vi "programa 4 Array.vi"() -> ()   [LabVIEW 2011]
panel:
  out "promedio":dbl
  out "menor":dbl
  out "mayor":dbl
  out "suma":dbl
  out "Array":dbl[](array[numeric])
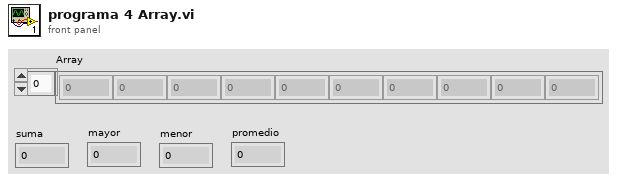
[diagram p1: front panel]
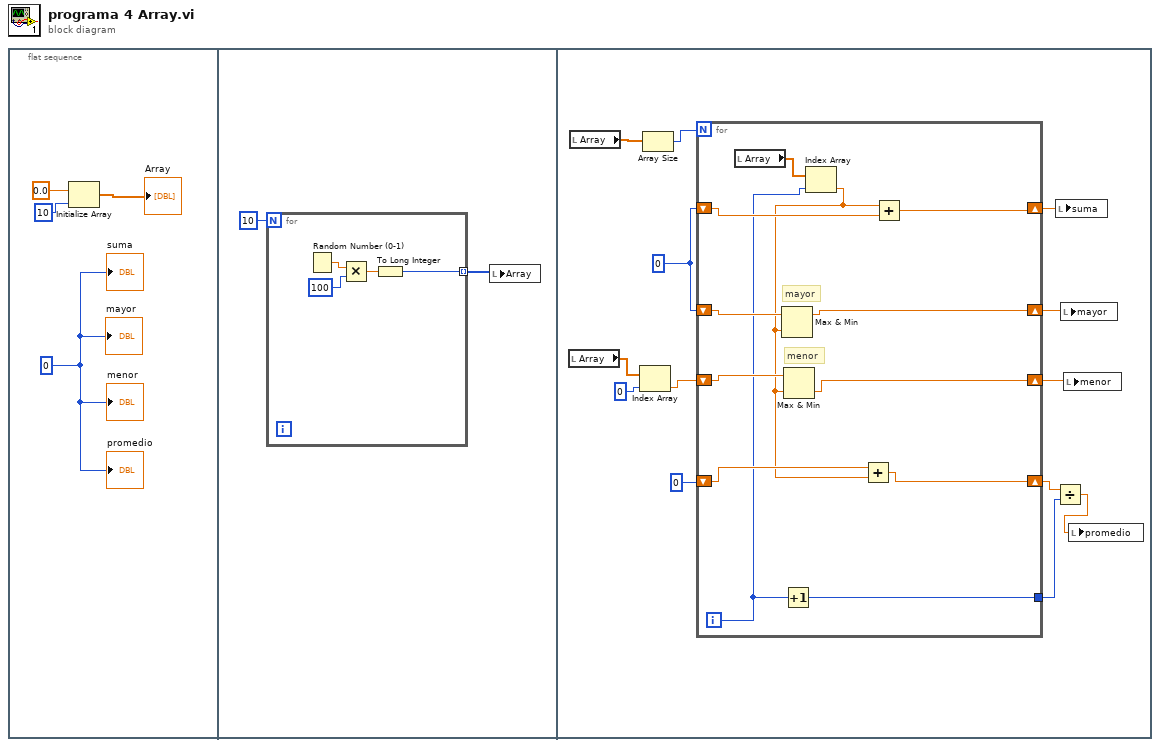
[diagram p0: block diagram]
diagram:
  n1 = flat-sequence {
    frame #0 {
      w1 = 0
      n2 = Initialize Array "Initialize Array"(0.0 ("element"), 10 ("dimension size")) -> (→"Array":dbl[])
      "suma" <- w1
      "mayor" <- w1
      "menor" <- w1
      "promedio" <- w1
    }
    frame #1 {
      n3 = for {
        N: 10 -> [_]
        tunnel: [w7] -> w5 mode=indexing
        n4 = Random Number (0-1)() -> (number: 0 to 1=w10:dbl)
        n5 = Multiply(x=w10, y=100) -> (x*y=w8:dbl)
        n6 = To Long Integer(number=w8) -> (32bit integer=w7:i32)
      }
      n7 = local write "Array"(w5) -> ()
    }
    frame #2 {
      w21 = 0
      n8 = local read "Array"() -> (w19:dbl[])
      n9 = local read "Array"() -> (w23:dbl[])
      n10 = Index Array(array=w19, index=0) -> (element=w17:dbl)
      n11 = Array Size(array=w23) -> (size(s)=w22:i32)
      n12 = for {
        N: w22 -> [_]
        shift-right: [w33] -> w20
        shift-left: w21 -> [w34]
        shift-right: [w29] -> w16
        shift-left: w21 -> [w32]
        shift-right: [w30] -> w15
        shift-left: w17 -> [w31]
        shift-right: [w26] -> w13
        shift-left: 0 -> [w28]
        tunnel: [w24] -> w12
        i -> [w25]
        # "menor"
        # "mayor"
        n13 = local read "Array"() -> (w35:dbl[])
        n14 = Increment(x=w25) -> (x+1=w24:i32)
        n15 = Index Array "Index Array"(array=w35, index=w25) -> (element=w27:dbl)
        n16 = Max & Min(x=w32, y=w27) -> (max(x,y)=w29:dbl)  [unwired: 1 out]
        n17 = Max & Min(x=w31, y=w27) -> (min(x,y)=w30:dbl)  [unwired: 1 out]
        n18 = Add(x=w28, y=w27) -> (x+y=w26:dbl)
        n19 = Add(x=w27, y=w34) -> (x+y=w33:dbl)
      }
      n20 = Divide(x=w13, y=w12) -> (x/y=w11:dbl)
      n21 = local write "suma"(w20) -> ()
      n22 = local write "mayor"(w16) -> ()
      n23 = local write "menor"(w15) -> ()
      n24 = local write "promedio"(w11) -> ()
    }
  }
